vi "core_binary_split_I32L.vi"(9 "vector in":i32[](array[numeric])) -> (0 "back":i32[](array[numeric]), 1 "middle":i32, 2 "front":i32[](array[numeric]), 4 "odd length?":bool)   [LabVIEW 2015]
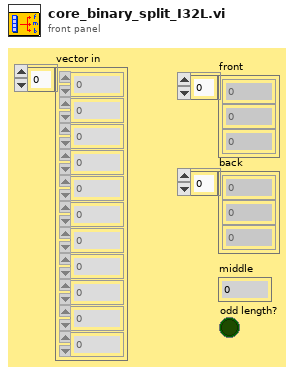
[diagram p1: front panel]
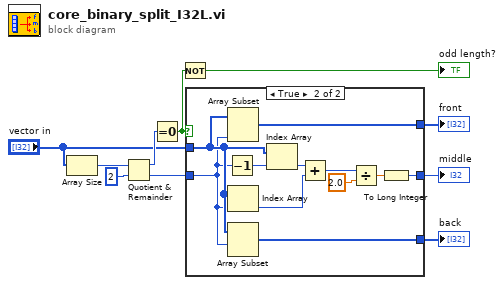
[diagram p0: block diagram]
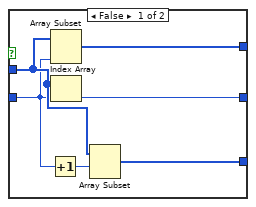
[diagram p2: hidden frame]
diagram:
  n1 = Array Size(array="vector in") -> (size(s)=w9:i32)
  n2 = Quotient & Remainder(x=w9, y=2) -> (x-y*floor(x/y)=w8:i32, floor(x/y)=w7:i32)
  n3 = Equal To 0?(x=w8) -> (x = 0?=w2:bool)
  n4 = Not(x=w2) -> (.not. x?=→"odd length?":bool)
  n5 = case shown="True" w2 {
    tunnel: "vector in" -> [w15 w25]
    tunnel: w7 -> [w14 w24]
    tunnel: [w13 w27] -> w5
    tunnel: [w12 w26] -> w4
    tunnel: [w11 w17] -> w3
    frame False {
      n6 = Increment(x=w14) -> (x+1=w16:i32)
      n7 = Array Subset(array=w15, length=w14) -> (w13:i32[])  [unwired: 1 in]
      n8 = Index Array(array=w15, index=w14) -> (element=w11:i32)
      n9 = Array Subset(array=w15, index=w16) -> (w12:i32[])  [unwired: 1 in]
    }
    frame True {
      n10 = Decrement(x=w24) -> (x-1=w23:i32)
      n11 = Array Subset(array=w25, length=w24) -> (w27:i32[])  [unwired: 1 in]
      n12 = Index Array(array=w25, index=w24) -> (element=w21:i32)
      n13 = Array Subset(array=w25, index=w24) -> (w26:i32[])  [unwired: 1 in]
      n14 = Index Array(array=w25, index=w23) -> (element=w22:i32)
      n15 = Add(x=w22, y=w21) -> (x+y=w20:i32)
      n16 = Divide(x=w20, y=2.0) -> (x/y=w18:dbl)
      n17 = To Long Integer(number=w18) -> (32bit integer=w17:i32)
    }
  }
  "front" <- w5
  "back" <- w4
  "middle" <- w3
